vi "Write DOM document.vi"(8 "error in":errorcluster, 10 "DOM document":refnum<k20>, 11 "System in":refnum<class "System.lvclass">) -> (0 "error out":errorcluster, 3 "System out":refnum<class "System.lvclass">)   [LabVIEW 2014, in "System.lvclass"]
uses:
  System.lvclass
  System.lvclass/System.ctl
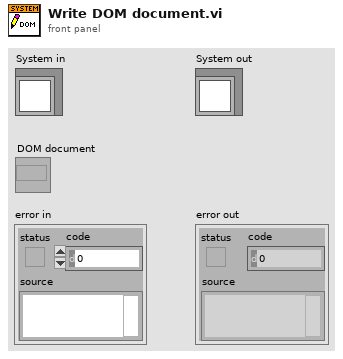
[diagram p1: front panel]
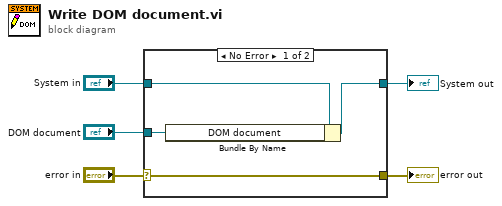
[diagram p0: block diagram]
diagram:
  n1 = case shown="No Error" "error in" {
    selector: "error in" -> [w9 w10]
    tunnel: [w9 w10] -> w4
    tunnel: [w7 w11] -> w2
    tunnel: "System in" -> [w8 w11]
    tunnel: "DOM document" -> [w6 _]
    frame No Error {
      n2 = Bundle By Name(cluster=w8, "DOM document"=w6) -> (w7:refnum<class "System.lvclass">)
    }
    frame Error {
    }
  }
  "error out" <- w4
  "System out" <- w2
